vi "get all lvlibp paths.vi"(8 "error in":errorcluster, 11 "Folder Path":path) -> (0 "error out":errorcluster, 3 "lvlibp path[]":path[](array[path]))   [LabVIEW 2020, in "Reusable Library.lvlib"]
doc: "Returns all lvlibp (packlibraries) from the specified folder recursively,\nIgnore folders or files staring with _ character"
uses:
  Reusable Library.lvlib
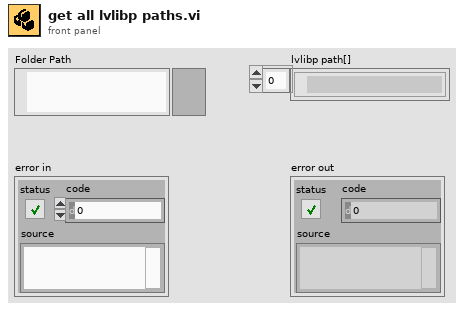
[diagram p1: front panel]
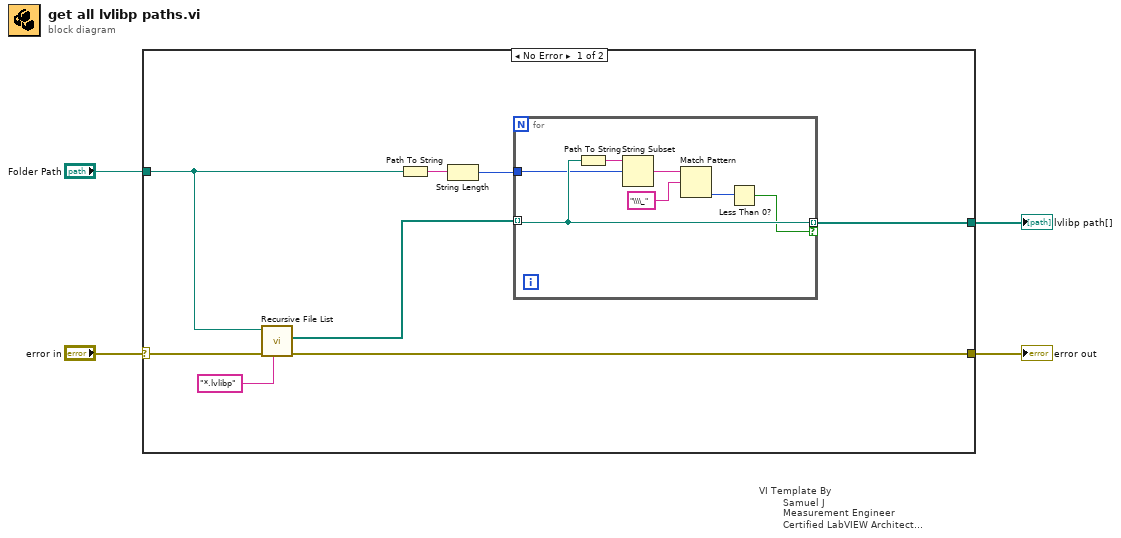
[diagram p0: block diagram]
diagram:
  n1 = case "VI Template By\n        Samuel J\n        Measurement Engineer\n        Certified LabVIEW Architect\n        Vestas Technology R&D Chennai" shown="No Error" "error in" {
    selector: "error in" -> [w6 w20]
    tunnel: "Folder Path" -> [w8 _]
    tunnel: [w7 _] -> w3
    tunnel: [w5 w20] -> w2
    frame No Error {
      n2 = call <vilib>:"Recursive File List.vi"("pattern"="*.lvlibp", "error in (no error)"=w6, "Folder Path"=w8) -> ("error out"=w5:errorcluster, "All Files in Dir"=w12:path[])  [unwired: 4 in, 3 out]
      n3 = Path To String(path=w8) -> (string=w10:string)
      n4 = String Length(string=w10) -> (length=w11:i32)
      n5 = for {
        tunnel: w12 -> [w19] mode=indexing
        tunnel: [w19] -> w7 mode=indexing if=w13
        tunnel: w11 -> [w17]
        n6 = Path To String(path=w19) -> (string=w18:string)
        n7 = String Subset(string=w18, offset (0)=w17) -> (substring=w16:string)  [unwired: 1 in]
        n8 = Match Pattern(string=w16, regular expression="\\\\_") -> (offset past match=w14:i32)  [unwired: 1 in, 3 out]
        n9 = Less Than 0?(x=w14) -> (x < 0?=w13:bool)
      }
    }
    frame Error {
    }
  }
  "lvlibp path[]" <- w3
  "error out" <- w2
